vi "Autonomous Independent.vi"   [LabVIEW 2014]
doc: "This VI is called when autonomous begins, and will automatically be terminated when autonomous ends. You can carry out timed or sensor driven robot movement independently without needing to return to the caller."
uses:
  <vilib>/Rock Robotics/WPI/Solenoid/WPI_SolenoidValue.ctl
  Robot Global Data.vi
  Auto Pickup Global.vi
  <vilib>/Rock Robotics/WPI/Solenoid/WPI_SolenoidSetEnum.vi
types:
  T1 = typedef "WPI_SolenoidValue.ctl" = enum16{"Off", "On", "Forward", "Reverse"}
  T2 = typedef "WPI_SolenoidDevRef.ctl" = cluster{"DevStatus":errorcluster, "Solenoid Module":T3, "Forward Solenoid Channel":T4, "Reverse Solenoid Channel":T4}
  T3 = typedef "FPGA_TypedefSolenoidModule.ctl" = enum16{"Solenoid Module 1", "Solenoid Module 2"}
  T4 = typedef "WPI_SolenoidChannel.ctl" = enum8{"Solenoid 1", "Solenoid 2", "Solenoid 3", "Solenoid 4", "Solenoid 5", "Solenoid 6", "Solenoid 7", "Solenoid 8", "Invalid"}
  T5 = typedef "Command Type.ctl" = cluster{"Function Name":string, "Arguments":string[]}
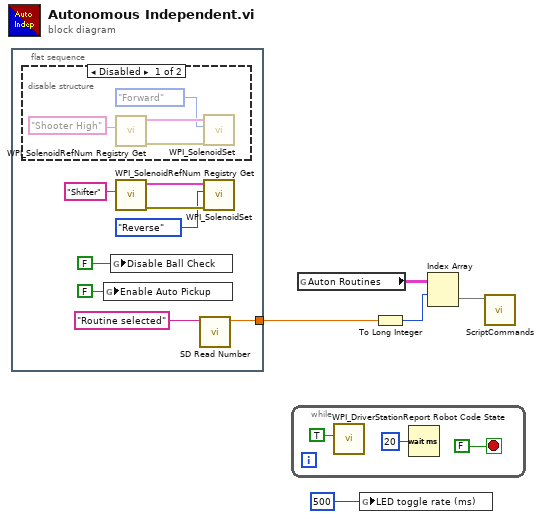
[diagram p0: block diagram]
diagram:
  n1 = flat-sequence {
    tunnel: [w10] -> w1
    frame #0 {
      n2 = disable-structure shown="Disabled" {
        frame Disabled {
          n3 = call <vilib>:"WPI_SolenoidRefNum Registry Get.vi"("refnum name"="Shooter High") -> ("error out"=w15:errorcluster, "SolenoidDevRef"=w16:T2)  [unwired: 9 in]
          n4 = call-poly <vilib>:"WPI_SolenoidSet.vi"("error in (no error)"=w15, "Value"=WPI_SolenoidValue."Forward", "SolenoidDevRef"=w16) -> ()  [unwired: 7 in, 2 out]
        }
        frame Enabled {
        }
      }
      n5 = global write "Auto Pickup Global.vi" "Enable Auto Pickup"(FALSE ("Enable Auto Pickup")) -> ()
      n6 = global write "Robot Global Data.vi" "Disable Ball Check"(FALSE ("Disable Ball Check")) -> ()
      n7 = call <vilib>:"WPI_SolenoidRefNum Registry Get.vi"("refnum name"="Shifter") -> ("error out"=w7:errorcluster, "SolenoidDevRef"=w8:T2)  [unwired: 9 in]
      n8 = call <vilib>:"SD Read Number.vi"("Name"="Routine selected") -> ("Numeric"=w10:dbl)  [unwired: 8 in, 2 out]
      n9 = call-poly <vilib>:"WPI_SolenoidSet.vi"("error in (no error)"=w7, "Value"=WPI_SolenoidValue."Reverse", "SolenoidDevRef"=w8) -> ()  [unwired: 7 in, 2 out]
    }
  }
  n10 = while {
    stop <- FALSE stop-if-true
    n11 = call <vilib>:"WPI_DriverStationReport Robot Code State.vi"("Autonomous"=TRUE) -> ()  [unwired: 10 in, 1 out]
    n12 = Wait (ms)(milliseconds to wait=u32 20) -> ()  [unwired: 1 out]
  }
  n13 = global read "Robot Global Data.vi" "Auton Routines"() -> (w3:T5[][])
  n14 = global write "Robot Global Data.vi" "LED toggle rate (ms)"(u32 500 ("LED ms toggle rate")) -> ()
  n15 = To Long Integer(number=w1) -> (32bit integer=w4:i32)
  n16 = Index Array(array=w3, index (row)=w4) -> (element=w2:T5[])  [unwired: 1 in]
  n17 = call "ScriptCommands.vi"("Auton Routines"=w2) -> ()  [unwired: 11 in]
